vi "gugudan server.vi"() -> ()   [LabVIEW 2014]
uses:
  <vilib>/FTP/NI_FTP.lvlib
panel:
  in  "숫자형":dbl min=0.0 max=24.0 format="%<%H:%M>t"
  in  "2시간":bool
  in  "재시작":bool
  in  "1시간":bool
  in  "강제종료":bool
  in  "종료취소":bool
  in  "종료":bool
  in  "사용설명서":bool
  out "로그인":bool
  in  "ID":string="ID"
  in  "PW":string="PW"
  in  "E-Mail":string="E-Mail  address"
  in  "명령전달":bool
  in  "address":string="ip address"
  out "참 거짓":string="상태창입니다."
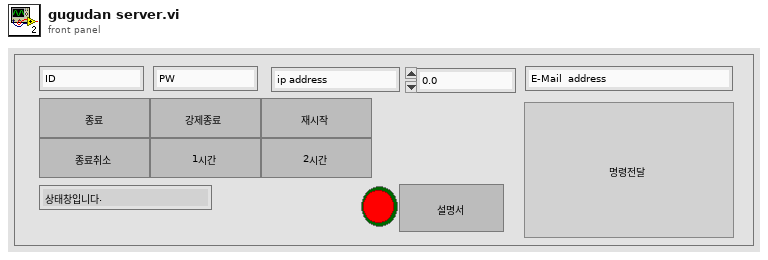
[diagram p1: front panel]
types:
  T1 = typedef "NI_FTP.lvlib/FTP Session.ctl" = refnum<k5>
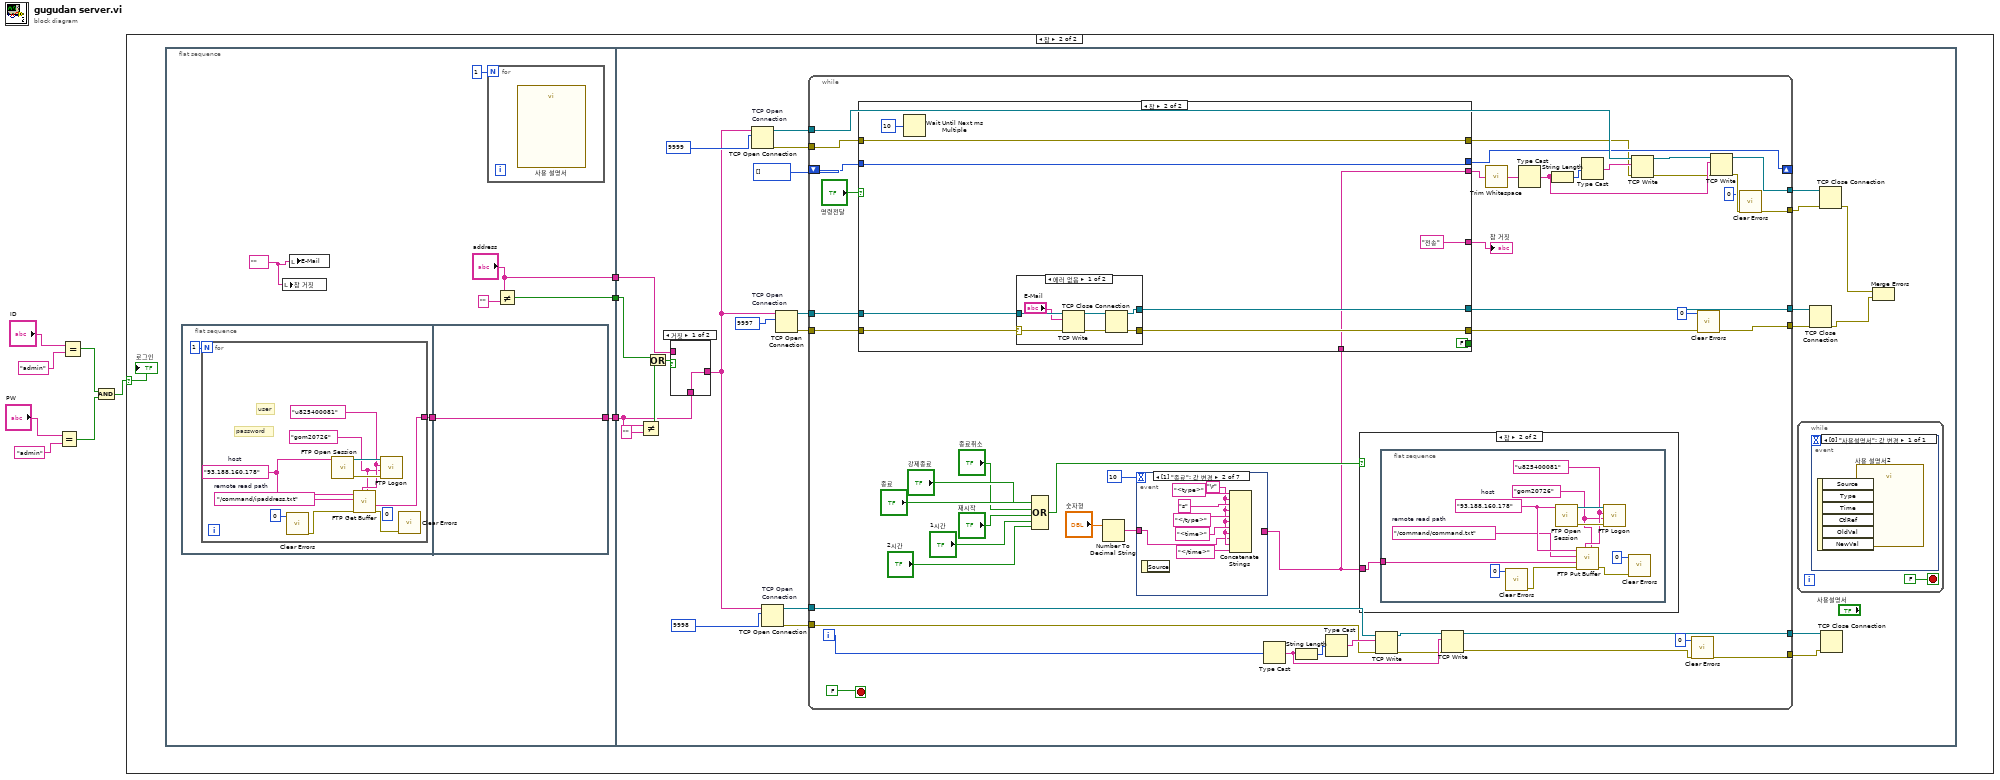
[diagram p0: block diagram]
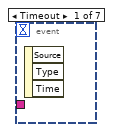
[diagram p5: hidden frame]
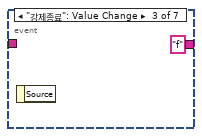
[diagram p6: hidden frame]
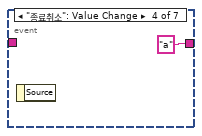
[diagram p7: hidden frame]
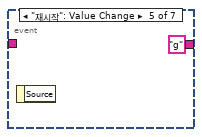
[diagram p8: hidden frame]
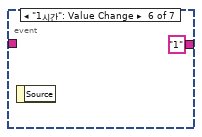
[diagram p9: hidden frame]
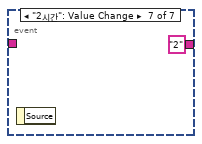
[diagram p10: hidden frame]
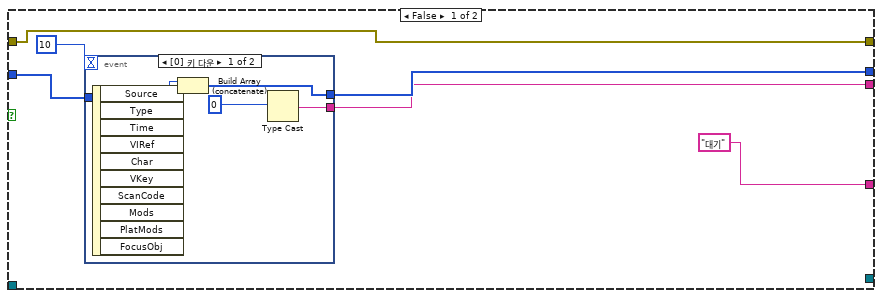
[diagram p11: hidden frame]
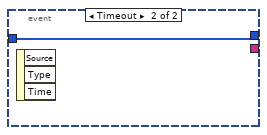
[diagram p12: hidden frame]
diagram:
  n1 = Equal?(x="PW", y="admin") -> (x = y?=w2:bool)
  n2 = Equal?(x="ID", y="admin") -> (x = y?=w3:bool)
  n3 = And(x=w3, y=w2) -> (x .and. y?=w1:bool)
  n4 = case shown="참" w1 {
    selector: w1 -> [_ w11]
    frame False {
    }
    frame True {
      n5 = flat-sequence {
        tunnel: [w17] -> w10
        tunnel: [w13] -> w9
        tunnel: ["address"] -> w8
        tunnel: w10 -> [w32]
        tunnel: w9 -> [w36]
        tunnel: w8 -> [w34]
        frame #0 {
          w15 = ""
          n6 = flat-sequence {
            tunnel: [w20] -> w16
            tunnel: [w31] -> w17
            tunnel: w16 -> [w31]
            frame #0 {
              n7 = for {
                N: 1 -> [_]
                tunnel: [w24] -> w20
                (unwired) 0 ("specific error code to clear (0: all)")
                w27 = "gom20726"
                w28 = "u825400081"
                w25 = "/command/ipaddress.txt"  # remote read path
                w26 = "93.188.160.178"  # host
                # "user"
                # "password"
                n8 = call <vilib>:"Clear Errors.vi"("specific error code to clear (0: all)"=0) -> ("error out"=w23:errorcluster)  [unwired: 5 in, 1 out]
                n9 = call <vilib>:"FTP Open Session.vi"("address"=w26) -> ("error out"=w29:errorcluster, "ftp session"=w30:T1)  [unwired: 7 in, 2 out]
                n10 = call <vilib>:"FTP Get Buffer.vi"("password"=w27, "user"=w28, "error in (no error)"=w23, "remote path"=w25, "host"=w26) -> ("error out"=w21:errorcluster, "data"=w24:string)  [unwired: 4 in, 1 out]
                n11 = call <vilib>:"FTP Logon.vi"("error in (no error)"=w29, "password"=w27, "user"=w28, "ftp session"=w30) -> ()  [unwired: 4 in, 4 out]
                n12 = call <vilib>:"Clear Errors.vi"("error in (no error)"=w21) -> ()  [unwired: 5 in, 2 out]
              }
            }
            frame #1 {
            }
          }
          n13 = local write "참 거짓"(w15) -> ()
          n14 = local write "E-Mail"(w15) -> ()
          n15 = for {
            N: 1 -> [_]
            n16 = call "사용 설명서"() -> ()  [unwired: 10 in, 2 out]
          }
          n17 = Not Equal?(x="address", y="") -> (x != y?=w13:bool)
        }
        frame #1 {
          n18 = Not Equal?(x=w32, y="") -> (x != y?=w37:bool)
          n19 = Or(x=w36, y=w37) -> (x .or. y?=w35:bool)
          n20 = case shown="거짓" w35 {
            tunnel: w34 -> [_ w58]
            tunnel: [w57 w58] -> w33
            tunnel: w32 -> [w57 _]
            frame False {
            }
            frame True {
            }
          }
          n21 = TCP Open Connection "TCP Open \nConnection"(address=w33, remote port or service name=u16 9999) -> (connection ID=w56:refnum<k5>, error out=w52:errorcluster)  [unwired: 3 in]
          n22 = TCP Open Connection "TCP Open \nConnection"(address=w33, remote port or service name=u16 9998) -> (connection ID=w49:refnum<k5>, error out=w46:errorcluster)  [unwired: 3 in]
          n23 = TCP Open Connection "TCP Open \nConnection"(address=w33, remote port or service name=u16 9997 ("원격 포트 또는 서비스 이름")) -> (connection ID=w44:refnum<k5>, error out=w43:errorcluster)  [unwired: 3 in]
          n24 = while {
            tunnel: w56 -> [w105]
            tunnel: [w107] -> w54
            shift-right: [w100] -> _
            shift-left: i16[] [] -> [w106]
            tunnel: w52 -> [w99]
            tunnel: [w79] -> w40
            tunnel: w49 -> [w87]
            tunnel: [w86] -> w48
            tunnel: [w76] -> w47
            tunnel: w46 -> [w85]
            tunnel: [w73] -> w45
            tunnel: w44 -> [w83]
            tunnel: w43 -> [w82]
            tunnel: [w81] -> w41
            i -> [w84]
            stop <- FALSE stop-if-true
            n25 = Compound Arithmetic op=OR("종료", "강제종료", "종료취소", "재시작", "1시간", "2시간") -> (w62:bool)
            n26 = Number To Decimal String(number="숫자형") -> (decimal integer string=w69:string)  [unwired: 1 in]
            n27 = event shown="[1] \"종료\": 값 변경" {
              selector: _ -> [_ _ _ _ _ _ _]
              dyn-events: _ -> [_ _ _ _ _ _ _]
              timeout: 10 -> [_ _ _ _ _ _ _]
              tunnel: w69 -> [_ w120 _ _ _ _ _]
              tunnel: [_ _ "f" "a" "g" "1" "2"] -> w60
              event Timeout {
                n28 = event-data() -> ()  [unwired: 1 in, 3 out]
              }
              event "종료": Value Change {
                w121 = "\r"
                n29 = event-data() -> ()  [unwired: 1 in, 1 out]
                n30 = Concatenate Strings("<type>", w121, "s", w121, "</type>", w121, "<time>", w121, w120, w121, "</time>") -> ()  [unwired: 1 out]
              }
              event "강제종료": Value Change {
                n31 = event-data() -> ()  [unwired: 1 in, 1 out]
              }
              event "종료취소": Value Change {
                n32 = event-data() -> ()  [unwired: 1 in, 1 out]
              }
              event "재시작": Value Change {
                n33 = event-data() -> ()  [unwired: 1 in, 1 out]
              }
              event "1시간": Value Change {
                n34 = event-data() -> ()  [unwired: 1 in, 1 out]
              }
              event "2시간": Value Change {
                n35 = event-data() -> ()  [unwired: 1 in, 1 out]
              }
            }
            n36 = case shown="참" "명령전달" {
              tunnel: w106 -> [w137 w153]
              tunnel: [w136 w153] -> w100
              tunnel: [w134 w144] -> w95
              tunnel: w99 -> [w133 w151]
              tunnel: [w133 w151] -> w98
              tunnel: ["대기" "전송"] -> w94
              tunnel: [_ FALSE ("불리언")] -> _
              tunnel: [_ w148] -> w72
              tunnel: w83 -> [_ w147]
              tunnel: w82 -> [_ w146]
              tunnel: [_ w145] -> w81
              tunnel: w60 -> [_ w144]
              frame False {
                n37 = event shown="[0] 키 다운" {
                  selector: _ -> [_ _]
                  dyn-events: _ -> [_ _]
                  timeout: 10 -> [_ _]
                  tunnel: [w141 w143] -> w136
                  tunnel: w137 -> [w142 w143]
                  tunnel: [w139 _] -> w134
                  event Key Down {
                    n38 = event-data() -> ("Char"=w140:i16)  [unwired: 1 in, 9 out]
                    n39 = Build Array (concatenate)(w140, w142) -> (w141:i16[])
                    n40 = Type Cast(x=0) -> (*(type *) &x=w139:string)  [unwired: 1 in]
                  }
                  event Timeout {
                    n41 = event-data() -> ()  [unwired: 1 in, 3 out]
                  }
                }
              }
              frame True {
                n42 = Wait Until Next ms Multiple(millisecond multiple=u32 10) -> ()  [unwired: 1 out]
                n43 = case shown="에러 없음" w146 {
                  selector: w146 -> [w155 w162]
                  tunnel: [w159 w161] -> w145
                  tunnel: [w158 w162] -> w148
                  tunnel: w147 -> [w156 w161]
                  frame No Error {
                    n44 = TCP Write(connection ID=w156, data in="E-Mail", error in (no error)=w155) -> (connection ID out=w160:refnum<k5>, error out=w157:errorcluster)  [unwired: 2 out]
                    n45 = TCP Close Connection(connection ID=w160, error in (no error)=w157) -> (connection ID out=w159:refnum<k5>, error out=w158:errorcluster)  [unwired: 1 out]
                  }
                  frame Error {
                  }
                }
              }
            }
            "참 거짓" <- w94
            n46 = Type Cast(x=w84) -> (*(type *) &x=w89:string)  [unwired: 1 in]
            n47 = String Length(string=w89) -> (length=w90:i32)
            n48 = Type Cast(x=w90) -> (*(type *) &x=w91:string)  [unwired: 1 in]
            n49 = case shown="참" w62 {
              tunnel: w60 -> [_ w108]
              frame False {
              }
              frame True {
                n50 = flat-sequence {
                  tunnel: w108 -> [w113]
                  frame #0 {
                    w116 = "gom20726"
                    w117 = "u825400081"
                    w114 = "/command/command.txt"  # remote read path
                    w115 = "93.188.160.178"  # host
                    n51 = call <vilib>:"Clear Errors.vi"("specific error code to clear (0: all)"=0) -> ("error out"=w111:errorcluster)  [unwired: 5 in, 1 out]
                    n52 = call <vilib>:"FTP Open Session.vi"("address"=w115) -> ("error out"=w118:errorcluster, "ftp session"=w119:T1)  [unwired: 7 in, 2 out]
                    n53 = call <vilib>:"FTP Put Buffer.vi"("password"=w116, "user"=w117, "error in (no error)"=w111, "data"=w113, "remote path"=w114, "host"=w115) -> ("error out"=w109:errorcluster)  [unwired: 4 in, 1 out]
                    n54 = call <vilib>:"FTP Logon.vi"("error in (no error)"=w118, "password"=w116, "user"=w117, "ftp session"=w119) -> ()  [unwired: 4 in, 4 out]
                    n55 = call <vilib>:"Clear Errors.vi"("error in (no error)"=w109, "specific error code to clear (0: all)"=0) -> ()  [unwired: 4 in, 2 out]
                  }
                }
              }
            }
            n56 = TCP Write(connection ID=w87, data in=w91, error in (no error)=w85) -> (connection ID out=w92:refnum<k5>, error out=w88:errorcluster)  [unwired: 1 in, 1 out]
            n57 = TCP Write(connection ID=w92, data in=w89, error in (no error)=w88) -> (connection ID out=w86:refnum<k5>, error out=w75:errorcluster)  [unwired: 1 in, 1 out]
            n58 = call <vilib>:"Trim Whitespace.vi"("string"=w95) -> ("trimmed string"=w96:string)  [unwired: 1 in]
            n59 = Type Cast(x=w96) -> (*(type *) &x=w101:string)  [unwired: 1 in]
            n60 = String Length(string=w101) -> (length=w102:i32)
            n61 = Type Cast(x=w102) -> (*(type *) &x=w103:string)  [unwired: 1 in]
            n62 = TCP Write(connection ID=w105, data in=w103, error in (no error)=w98) -> (connection ID out=w104:refnum<k5>, error out=w97:errorcluster)  [unwired: 1 in, 1 out]
            n63 = call <vilib>:"Clear Errors.vi"("error in (no error)"=w75, "specific error code to clear (0: all)"=0) -> ("error out"=w76:errorcluster)  [unwired: 4 in, 1 out]
            n64 = call <vilib>:"Clear Errors.vi"("error in (no error)"=w72, "specific error code to clear (0: all)"=0) -> ("error out"=w73:errorcluster)  [unwired: 4 in, 1 out]
            n65 = TCP Write(connection ID=w104, data in=w101, error in (no error)=w97) -> (connection ID out=w107:refnum<k5>, error out=w78:errorcluster)  [unwired: 1 in, 1 out]
            n66 = call <vilib>:"Clear Errors.vi"("error in (no error)"=w78, "specific error code to clear (0: all)"=0) -> ("error out"=w79:errorcluster)  [unwired: 4 in, 1 out]
          }
          n67 = while {
            stop <- FALSE stop-if-true
            n68 = event shown="[0] \"사용설명서\": 값 변경" {
              selector: _ -> [_]
              dyn-events: _ -> [_]
              timeout: _ -> [_]
              event "사용설명서": Value Change {
                n69 = event-data() -> ()  [unwired: 1 in, 6 out]
                n70 = call "사용 설명서2"() -> ()  [unwired: 10 in, 2 out]
              }
            }
          }
          n71 = TCP Close Connection(connection ID=w41, error in (no error)=w45) -> (error out=w39:errorcluster)  [unwired: 2 out]
          n72 = TCP Close Connection(connection ID=w54, error in (no error)=w40) -> (error out=w51:errorcluster)  [unwired: 1 in, 1 out]
          n73 = TCP Close Connection(connection ID=w48, error in (no error)=w47) -> ()  [unwired: 1 in, 2 out]
          n74 = Merge Errors(w51, w39) -> ()  [unwired: 1 out]
        }
      }
      "로그인" <- w11
    }
  }
